vi "P541_Quit.vi"(11 "VISA Refnum in":refnum<visa-resource-name>) -> ()   [LabVIEW 2011]
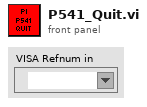
[diagram p1: front panel]
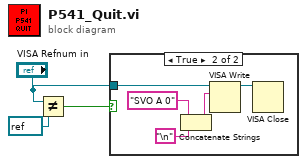
[diagram p0: block diagram]
diagram:
  n1 = Not Equal?(x="VISA Refnum in", y=refnum<visa-resource-name> refnum ("VISA resource name")) -> (x != y?=w1:bool)
  n2 = case shown="True" w1 {
    tunnel: "VISA Refnum in" -> [_ w8]
    frame False {
    }
    frame True {
      n3 = Concatenate Strings("SVO A 0" ("write buffer"), "\n") -> (w5:string)
      n4 = VISA Write(VISA resource name=w8, write buffer=w5) -> (VISA resource name out=w7:refnum<visa-resource-name>)  [unwired: 1 in, 2 out]
      n5 = VISA Close(VISA resource name=w7) -> ()  [unwired: 1 in, 1 out]
    }
  }
